vi "test Add Connections.vi"(8 "error in (no error)":errorcluster, 11 "TestCase in":refnum<class "Switch Scripting Test Case.lvclass">) -> (0 "error out":errorcluster, 3 "TestCase out":refnum<class "Switch Scripting Test Case.lvclass">)   [LabVIEW 2017, in "Switch Scripting.lvlib" / "Switch Scripting Test Case.lvclass"]
uses:
  Switch Scripting Test Case.lvclass
  Routing Channel/Connection.ctl
  Routing State.ctl
  Switch Scripting Test Case.lvclass/Switch Scripting Test Case.ctl
  <vilib>/addons/_JKI Toolkits/VI Tester/TestCase.llb/TestCase.lvclass
  Switch Scripting.lvlib
  C:/Program Files (x86)/National Instruments/LabVIEW 2017/vi.lib/addons/_JKI Toolkits/VI Tester/TestCase.llb/TestCase.lvclass
panel:
  in  "Save?":bool
  out "Output Filename":string
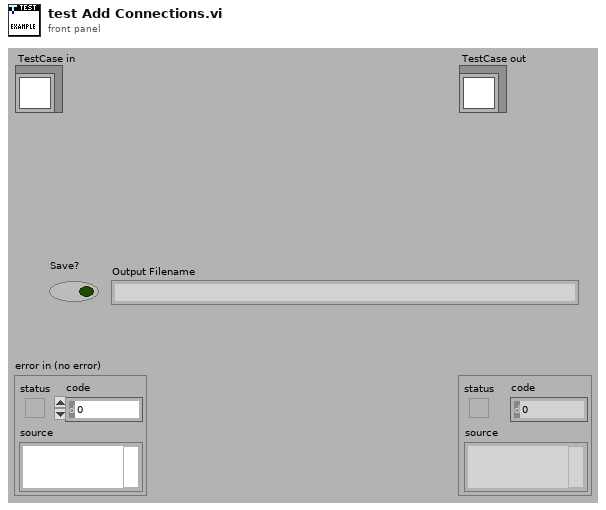
[diagram p1: front panel]
types:
  T1 = typedef "Switch Scripting.lvlib/Routing State.ctl" = cluster{"name":string, "description":string, "value":i32, "connection list":T2[]}
  T2 = typedef "Switch Scripting.lvlib/Connection.ctl" = cluster{"source":string, "destination":string}
  T3 = typedef "Custom Device API.lvlib/Custom Device Item Ref.ctl" = u64
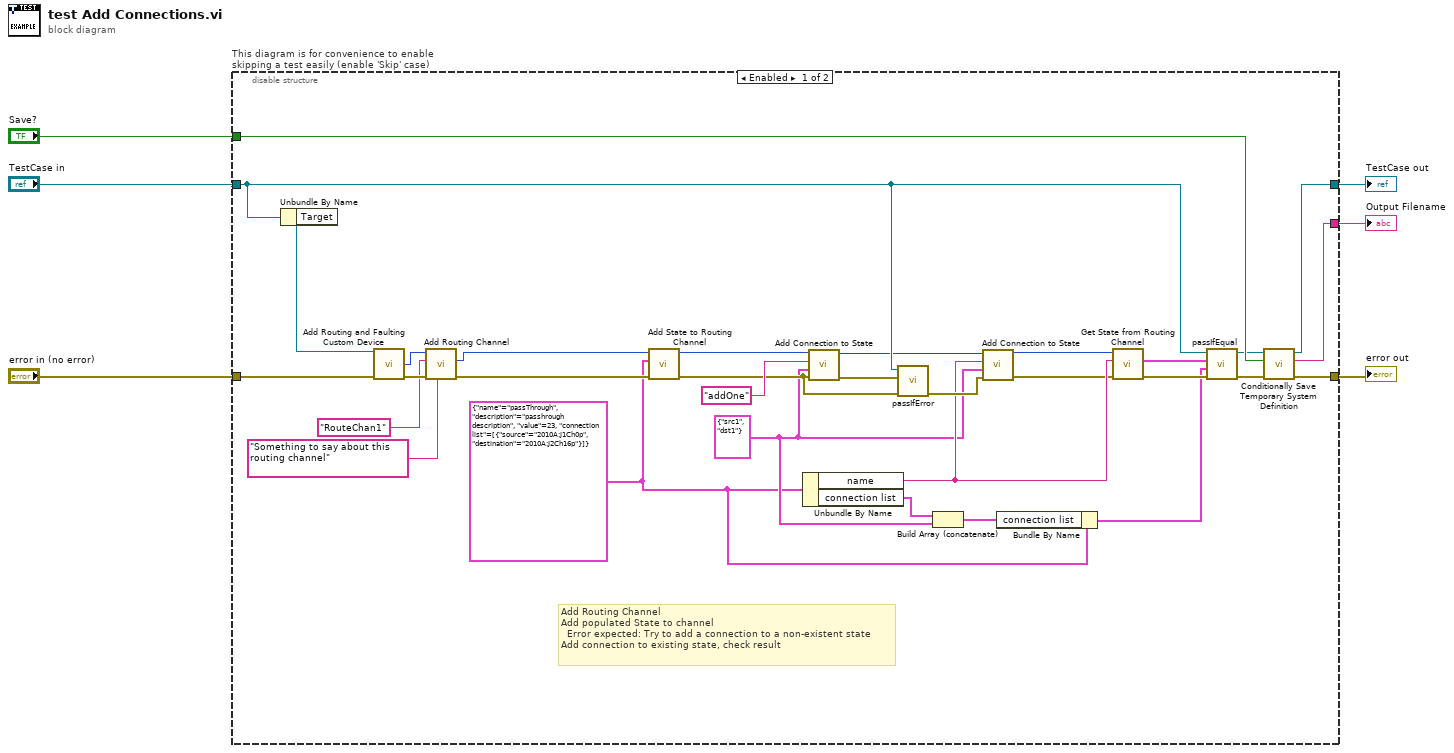
[diagram p0: block diagram]
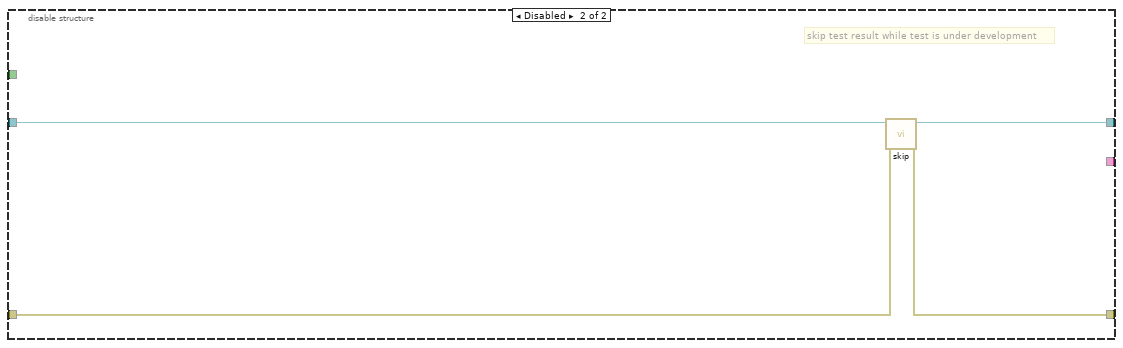
[diagram p2: hidden frame]
diagram:
  n1 = disable-structure "This diagram is for convenience to enable skipping a test easily (enable 'Skip' case)" shown="Enabled" {
    disable-tunnel: "TestCase in" -> [w21 w41]
    disable-tunnel: [w32 w39] -> w3
    disable-tunnel: [w36 w40] -> w5
    disable-tunnel: "error in (no error)" -> [w37 w38]
    disable-tunnel: [w35 _] -> w2
    disable-tunnel: "Save?" -> [w34 _]
    frame Enabled {
      w9 = T1 {"name"="passThrough", "description"="passhrough description", "value"=23, "connection list"=[{"source"="2010A:J1Ch0p", "destination"="2010A:J2Ch16p"}]} ("Routing State")
      w10 = T2 {"source"="src1", "destination"="dst1"} ("connection")
      # "Add Routing Channel\nAdd populated State to channel\n  Error expected: Try to add a connection to a non-existent state\nAdd connection to existing state, check result"
      n2 = Unbundle By Name(w21) -> ("Target"=w33:refnum<k24>)
      n3 = call "Add Routing and Faulting Custom Device.vi"("Target in"=w33, "error in (no error)"=w37) -> ("Routes Section Ref"=w27:T3, "error out"=w31:errorcluster)  [unwired: 9 in, 3 out]
      n4 = call "Add Routing Channel.vi"("Description"="Something to say about this routing channel", "error in (no error)"=w31, "Channel Name"="RouteChan1", "Routes Ref in"=w27) -> ("error out"=w22:errorcluster, "Channel Ref"=w18:T3)  [unwired: 5 in, 1 out]
      n5 = call "Add State to Routing Channel.vi"("error in (no error)"=w22, "Routing State"=w9, "Channel Ref in"=w18) -> ("error out"=w19:errorcluster, "Channel Ref out"=w17:T3)  [unwired: 7 in]
      n6 = Unbundle By Name(w9) -> ("name"=w14:string, "connection list"=w11:T2[])
      n7 = call "Add Connection to State.vi"("error in (no error)"=w19, "Connection"=w10, "State"="addOne" ("state name"), "Channel Ref in"=w17) -> ("error out"=w20:errorcluster, "Channel Ref out"=w16:T3)  [unwired: 6 in]
      n8 = call-dynamic "passIfError.vi"("error in (no error)"=w19, "error"=w20, "TestCase in"=w21) -> ("error out"=w15:errorcluster)  [unwired: 7 in, 1 out]
      n9 = Build Array (concatenate)(w11, w10) -> (w8:T2[])
      n10 = call "Add Connection to State.vi"("error in (no error)"=w15, "Connection"=w10, "State"=w14, "Channel Ref in"=w16) -> ("error out"=w12:errorcluster, "Channel Ref out"=w13:T3)  [unwired: 6 in]
      n11 = Bundle By Name(cluster=w9, "connection list"=w8) -> (w7:T1)
      n12 = call "Get State from Routing Channel.vi"("error in (no error)"=w12, "State"=w14, "Channel Ref in"=w13) -> ("error out"=w26:errorcluster, "Routing State"=w25:T1)  [unwired: 6 in, 1 out]
      n13 = call-dynamic "passIfEqual.vi"("error in (no error)"=w26, "y"=w7, "x"=w25, "TestCase in"=w21) -> ("error out"=w30:errorcluster, "TestCase out"=w29:refnum<class "Switch Scripting Test Case.lvclass">)  [unwired: 6 in]
      n14 = call "Conditionally Save Temporary System Definition.vi"("error in (no error)"=w30, "Save?"=w34, "Test Case"=w29) -> ("error out"=w36:errorcluster, "filename"=w35:string, "Test Case"=w32:refnum<class "Switch Scripting Test Case.lvclass">)  [unwired: 6 in]
    }
    frame Disabled {
      # "skip test result while test is under development"
      n15 = call <vilib>:"skip.vi"("error in (no error)"=w38, "TestCase in"=w41) -> ("error out"=w40:errorcluster, "TestCase out"=w39:refnum<class "Switch Scripting Test Case.lvclass">)  [unwired: 8 in]
    }
  }
  "error out" <- w5
  "TestCase out" <- w3
  "Output Filename" <- w2
